vi "Autonomous Independent.vi"   [LabVIEW 2020]
doc: "This VI is called when autonomous begins, and will automatically be terminated when autonomous ends. You can carry out timed or sensor driven robot movement independently without needing to return to the caller."
uses:
  <vilib>/Rock Robotics/WPI/Utilities/WPI_GetSetVariantRefNum.vi
  Robot Global Data.vi
  <vilib>/Rock Robotics/Network Tables/NT Read Number.vi
  <vilib>/Rock Robotics/Network Tables/NT Write Numeric Array.vi
  <vilib>/Rock Robotics/Network Tables/NT Read String.vi
panel:
  # "Be sure to right-click and choose Data Operations>>Make Current Value default if you want to save the array values with the VI"
types:
  T1 = typedef "WPI_JoystickDevRef.ctl" = cluster{"Device":T2}
  T2 = typedef "WPI_JoystickDeviceEnum.ctl" = enum16{"USB 0", "USB 1", "USB 2", "USB 3", "USB 4", "USB 5"}
  T3 = typedef "WPI_MotorControlDeviceRef.ctl" = cluster{"DeviceStatus":errorcluster, "Type":T4, "PWM":cluster{"PWM Channel":T5, "DeadBand":T6}, "CAN":cluster{"Device Number":u8, "SetOutput VI Ref":variant, "GetOutput VI Ref":variant, "Enable VI Ref":variant, "Disable VI Ref":variant, "Data":variant}, "Invert":bool, "DIO PWM":cluster{"PWM \"Enable\" Channel":T5, "DIOChannel":T7, "PWM Rate":dbl}}
  T4 = typedef "WPI_MotorControlType.ctl" = enum16{"PWM", "CAN", "DIO PWM"}
  T5 = typedef "FPGA_DIOPWMChannel.ctl" = enum8{"PWM 0", "PWM 1", "PWM 2", "PWM 3", "PWM 4", "PWM 5", "PWM 6", "PWM 7", "PWM 8", "PWM 9", "PWM MXP 0", "PWM MXP 1", "PWM MXP 2", "PWM MXP 3", "PWM MXP 4", "PWM MXP 5", "PWM MXP 6", "PWM MXP 7", "PWM MXP 8", "PWM MXP 9", "Invalid"}
  T6 = typedef "WPI_PWMDeadband.ctl" = cluster{"Name":string, "maxPositivePwm":i32, "minPositivePwm":i32, "centerPwm":i32, "maxNegativePwm":i32, "minNegativePwm":i32, "angularRange":u16}
  T7 = typedef "FPGA_DIOChannel.ctl" = enum8{"DIO 0", "DIO 1", "DIO 2", "DIO 3", "DIO 4", "DIO 5", "DIO 6", "DIO 7", "DIO 8", "DIO 9", "DIO MXP 0", "DIO MXP 1", "DIO MXP 2", "DIO MXP 3", "DIO MXP 4", "DIO MXP 5", "DIO MXP 6", "DIO MXP 7", "DIO MXP 8", "DIO MXP 9", "DIO MXP 10", "DIO MXP 11", "DIO MXP 12", "DIO MXP 13", "DIO MXP 14", "DIO MXP 15", "SPI Port CS1", "SPI Port CS2", "SPI Port CS3", "SPI Port MISO", "SPI Port MOSI", "Invalid"}
  T8 = typedef "WPI_RobotDriveDevRef.ctl" = cluster{"DevStatus":errorcluster, "Motors[]":T3[], "Square Inputs":bool, "Max Output":dbl}
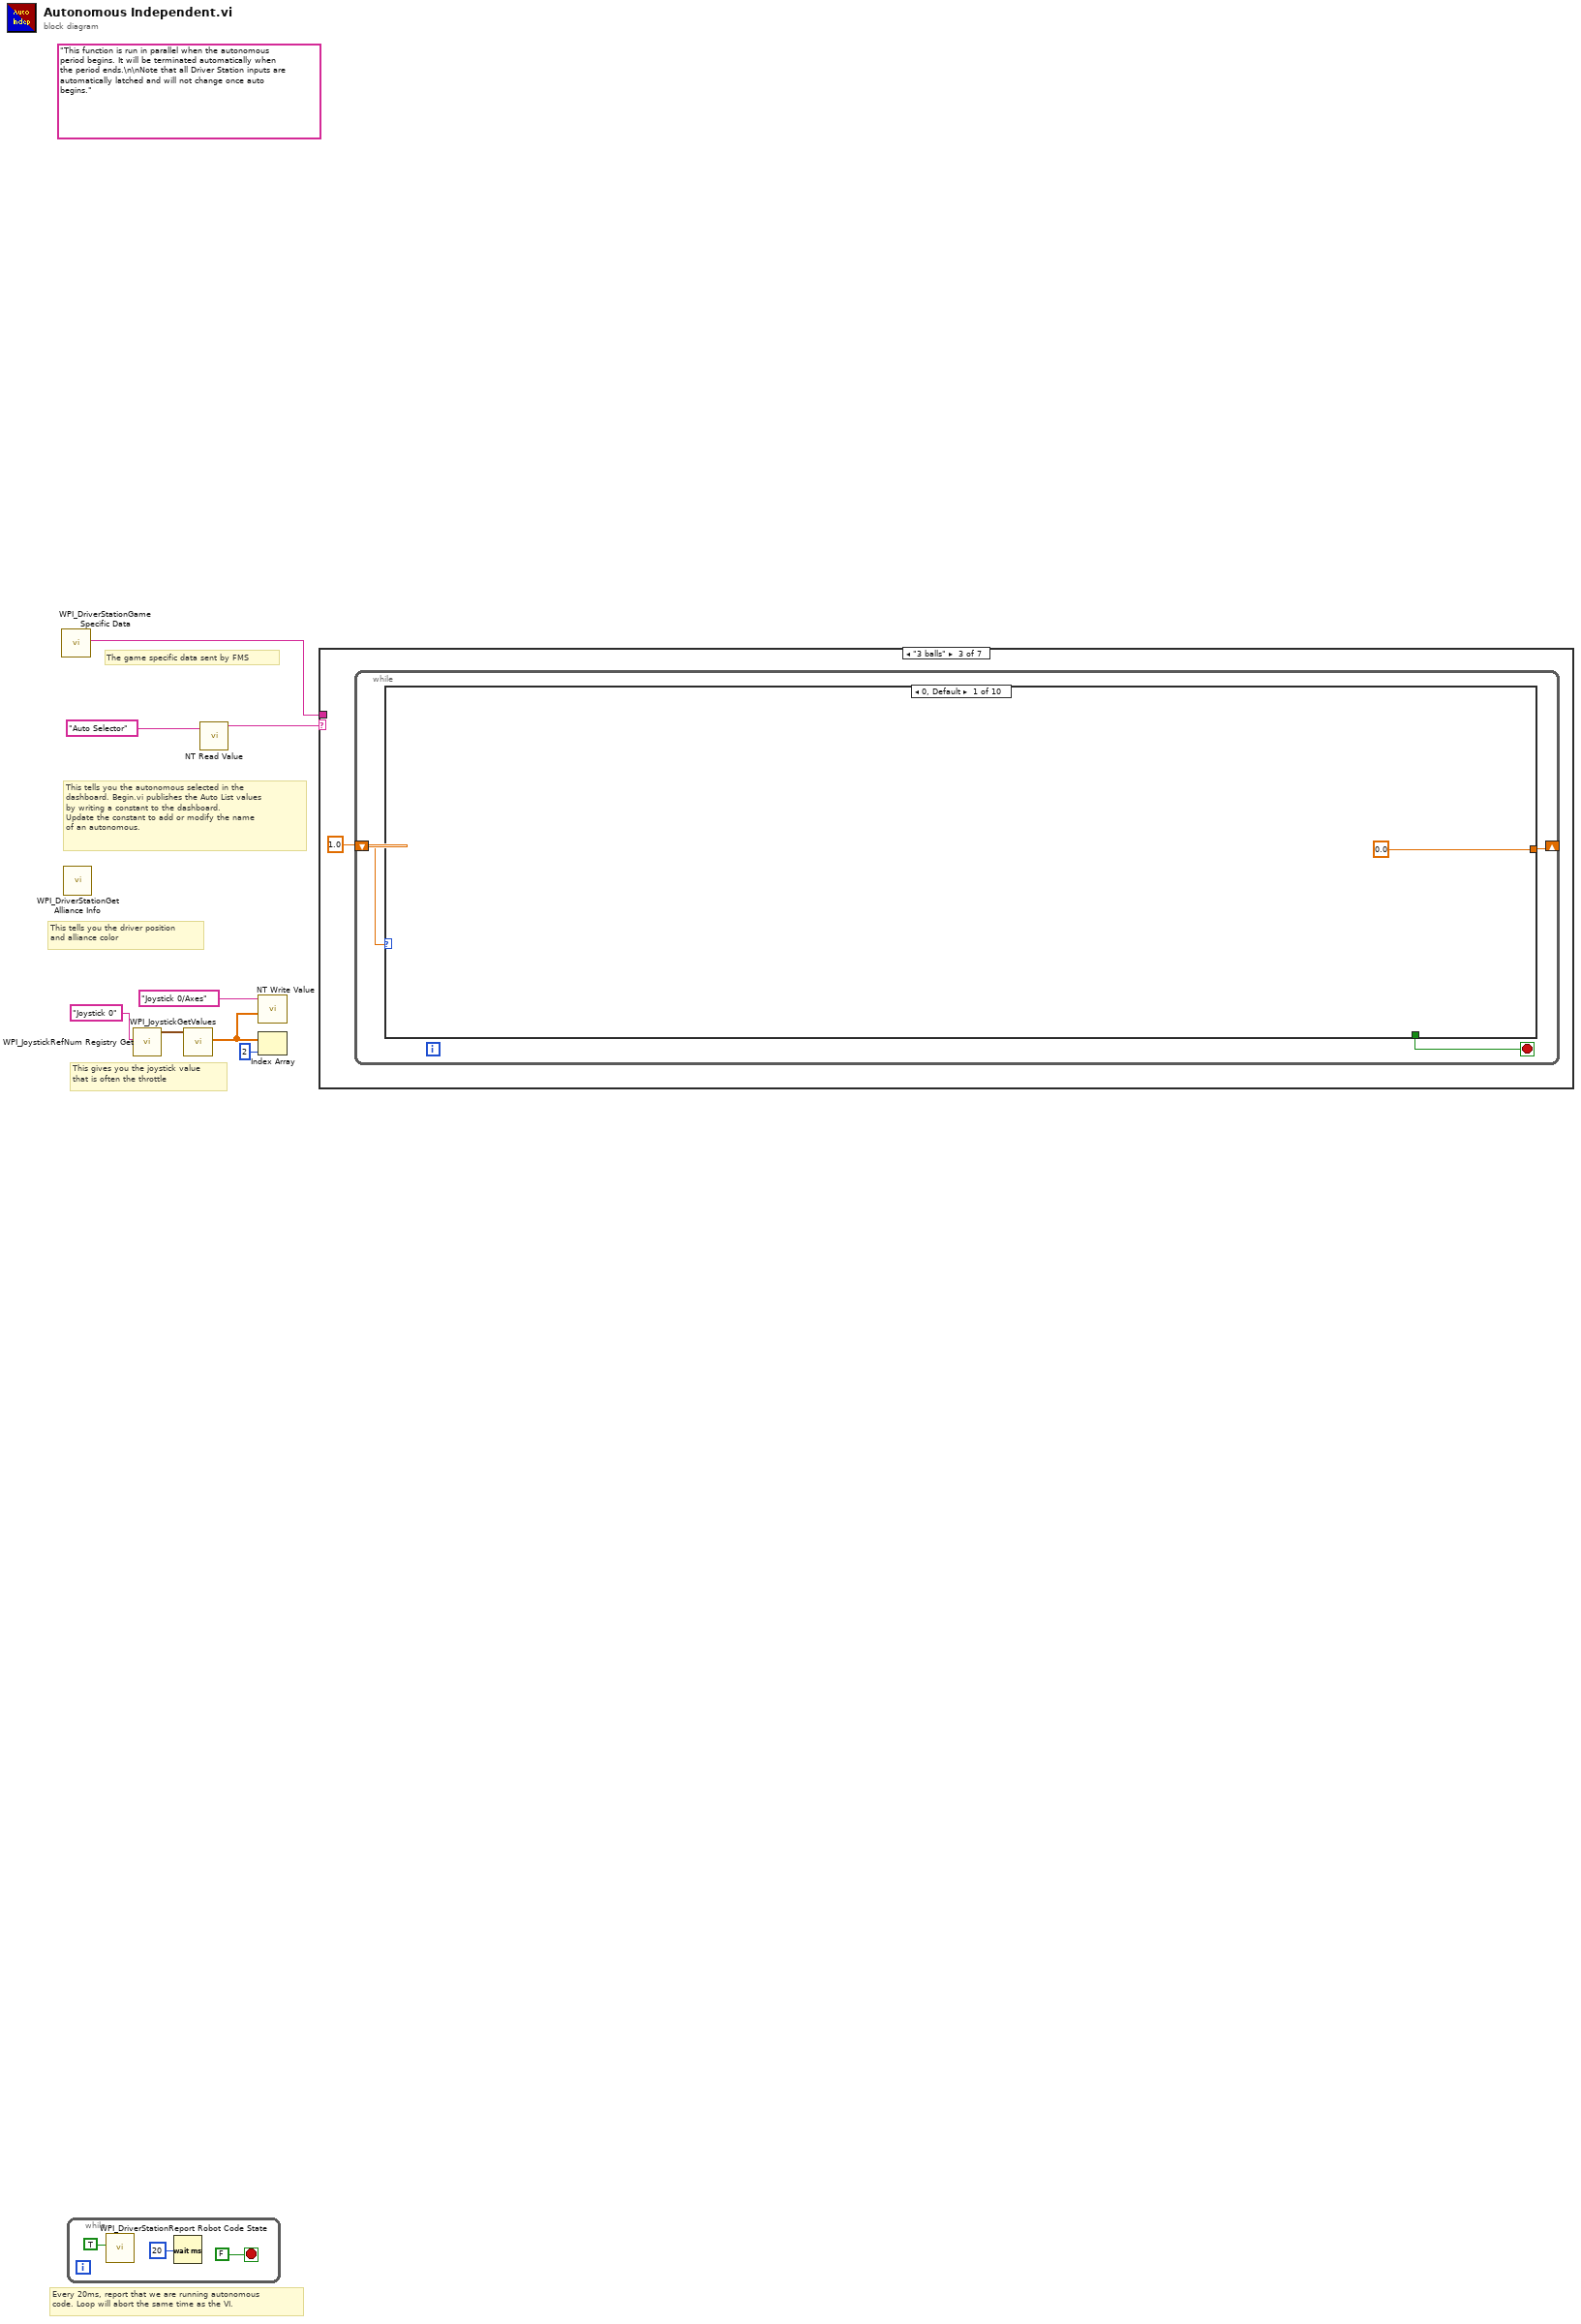
[diagram p0: block diagram]
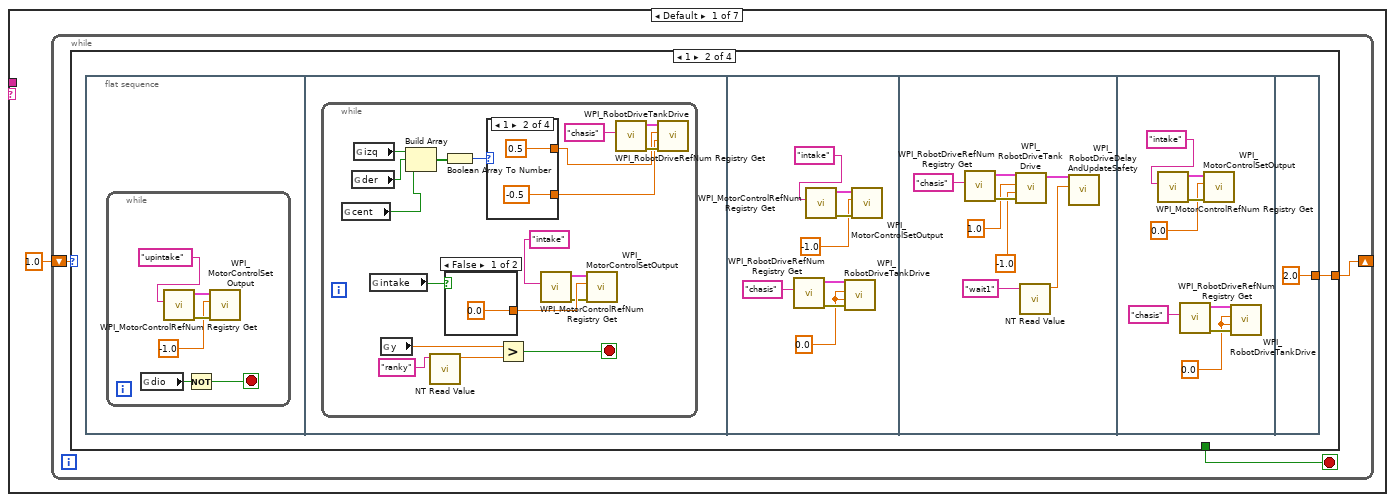
[diagram p2: hidden frame]
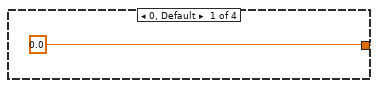
[diagram p3: hidden frame]
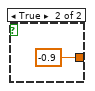
[diagram p4: hidden frame]
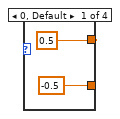
[diagram p5: hidden frame]
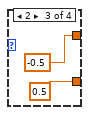
[diagram p6: hidden frame]
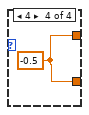
[diagram p7: hidden frame]
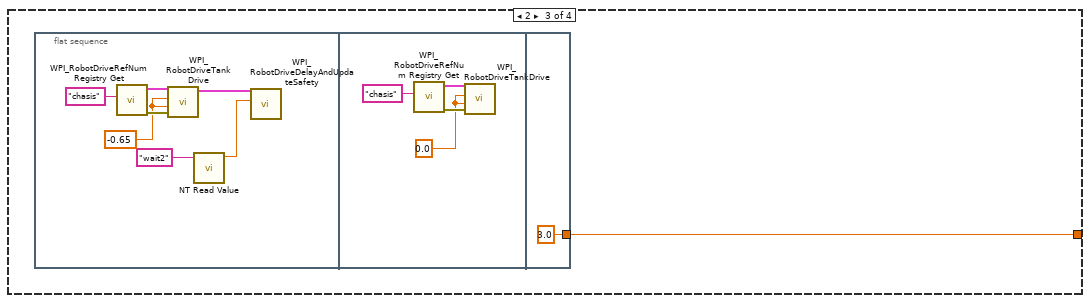
[diagram p8: hidden frame]
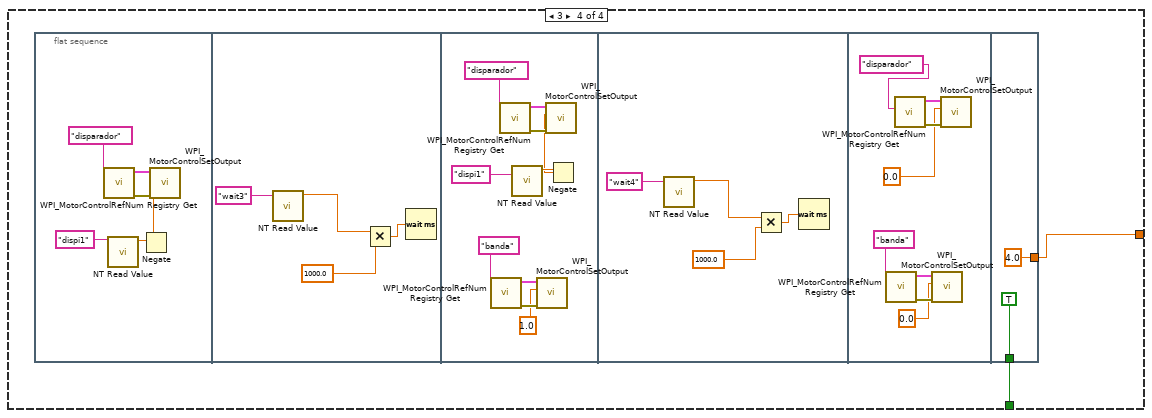
[diagram p9: hidden frame]
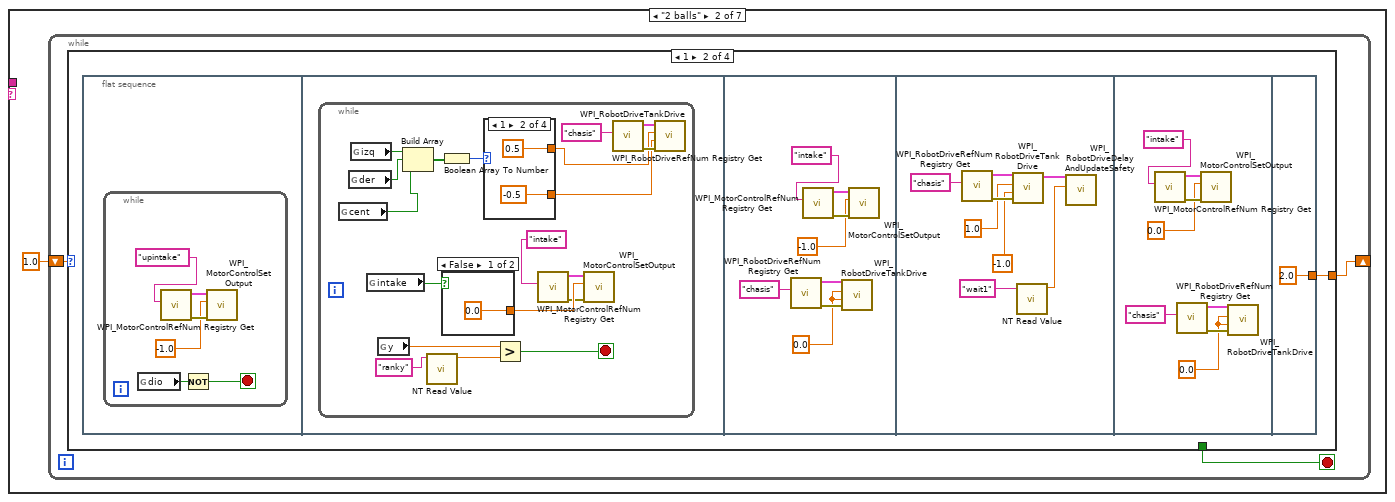
[diagram p10: hidden frame]
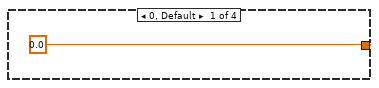
[diagram p11: hidden frame]
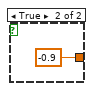
[diagram p12: hidden frame]
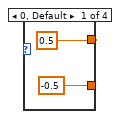
[diagram p13: hidden frame]
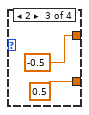
[diagram p14: hidden frame]
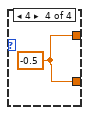
[diagram p15: hidden frame]
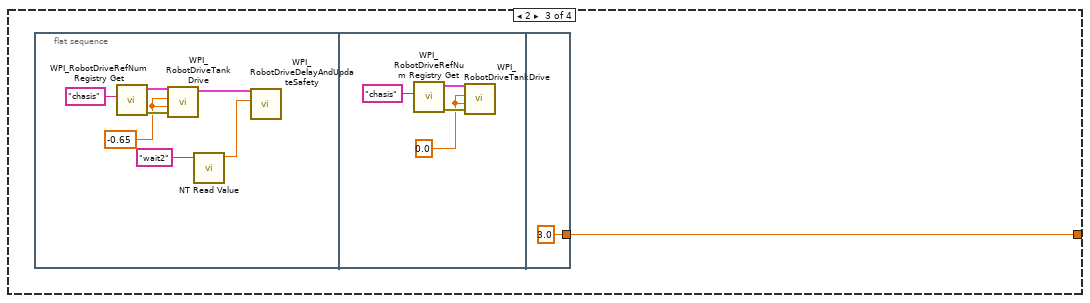
[diagram p16: hidden frame]
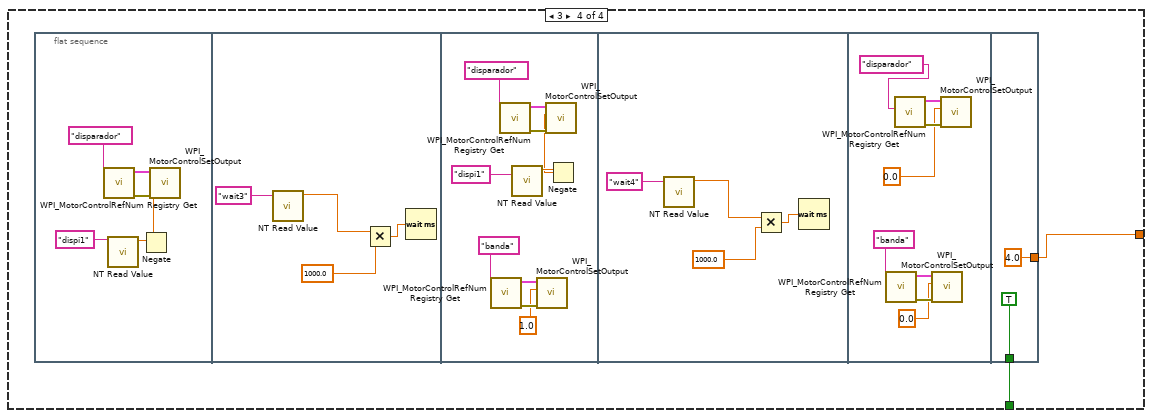
[diagram p17: hidden frame]
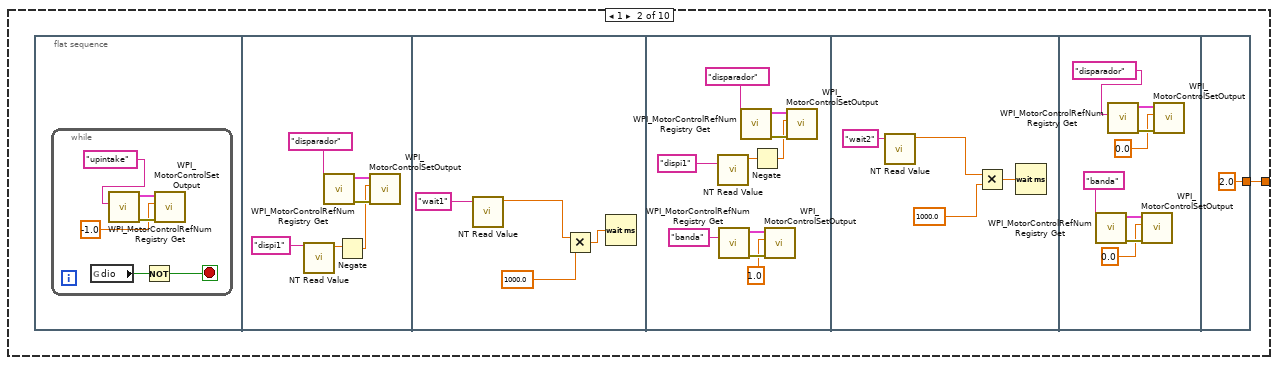
[diagram p18: hidden frame]
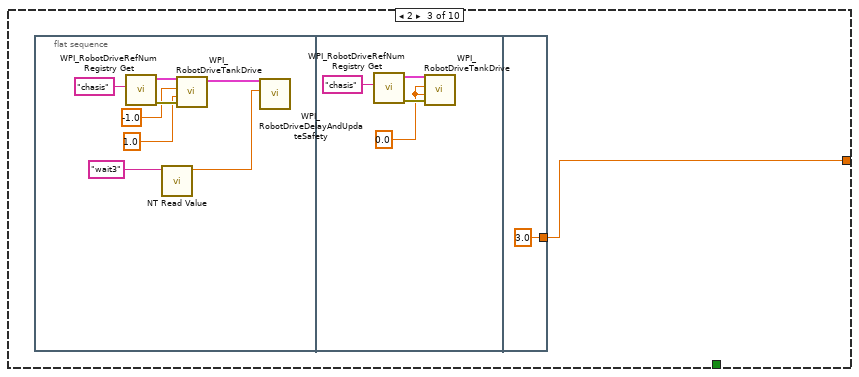
[diagram p19: hidden frame]
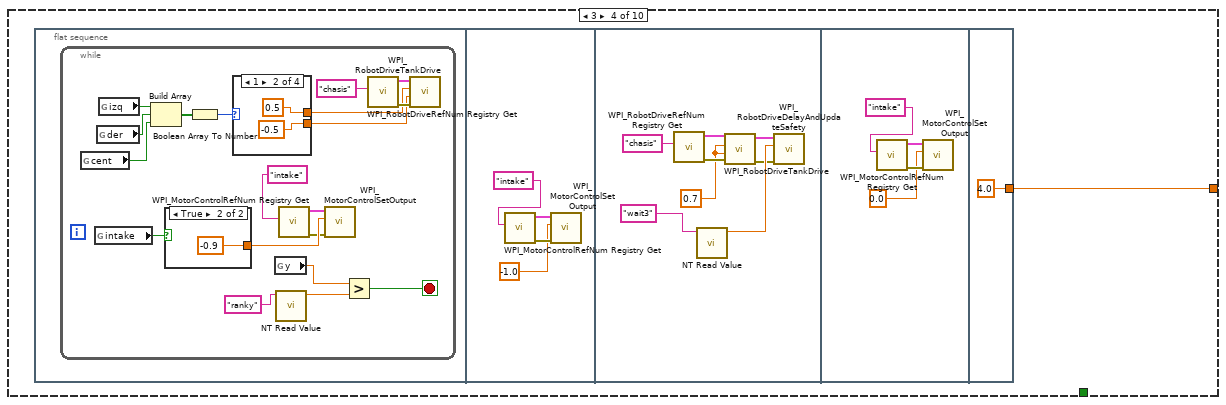
[diagram p20: hidden frame]
diagram:
  (unwired) "This function is run in parallel when the autonomous period begins. It will be terminated automatically when the period ends.\n\nNote that all Driver Station inputs are automatically latched and will not change once auto begins."
  # "The game specific data sent by FMS"
  # "This tells you the autonomous selected in the \ndashboard. Begin.vi publishes the Auto List values\nby writing a constant to the dashboard.\nUpdate the constant to add or modify the name\nof an autonomous."
  # "Every 20ms, report that we are running autonomous\ncode. Loop will abort the same time as the VI."
  # "This gives you the joystick value\nthat is often the throttle"
  # "This tells you the driver position\nand alliance color"
  n1 = call <vilib>:"WPI_DriverStationGame Specific Data.vi"() -> ("Game Specific Data"=w1:string)  [unwired: 11 in]
  n2 = call <vilib>:"WPI_DriverStationGet Alliance Info.vi"() -> ()  [unwired: 12 out]
  n3 = while {
    stop <- FALSE stop-if-true
    n4 = call <vilib>:"WPI_DriverStationReport Robot Code State.vi"("Autonomous"=TRUE) -> ()  [unwired: 10 in, 1 out]
    n5 = Wait (ms)(milliseconds to wait=u32 20) -> ()  [unwired: 1 out]
  }
  n6 = call <vilib>:"WPI_JoystickRefNum Registry Get.vi"("refnum name"="Joystick 0") -> ("JoystickDevRef"=w7:T1)  [unwired: 1 in, 9 out]
  n7 = call <vilib>:"WPI_JoystickGetValues.vi"("JoystickDevRef"=w7) -> ("Axes"=w3:dbl[])  [unwired: 6 in, 4 out]
  n8 = call-poly <vilib>:"NT Read Value.vi"("Name"="Auto Selector") -> ("String"=w4:string)  [unwired: 9 in, 1 out]
  n9 = call-poly <vilib>:"NT Write Value.vi"("Numeric Array"=w3, "Name"="Joystick 0/Axes") -> ()  [unwired: 9 in, 1 out]
  n10 = Index Array(array=w3, index=2) -> ()  [unwired: 1 out]
  n11 = case shown="\"3 balls\"" w4 {
    tunnel: w1 -> [_ _ _ _ _ _ _]
    frame Default {
      n12 = while {
        shift-right: [w14] -> _
        shift-left: 1.0 -> [w15]
        stop <- w13 stop-if-true
        n13 = case shown="1" w15 {
          tunnel: [0.0 w17 w77 w90] -> w14
          tunnel: [_ _ _ w91] -> w13
          frame 0, Default {
          }
          frame 1 {
            n14 = flat-sequence {
              tunnel: [2.0] -> w17
              frame #0 {
                n15 = while {
                  stop <- w18 stop-if-true
                  n16 = global read "Robot Global Data.vi" "dio"() -> (w19:bool)
                  n17 = call <vilib>:"WPI_MotorControlRefNum Registry Get.vi"("refnum name"="upintake") -> ("error out"=w22:errorcluster, "MotorControlDevRef"=w23:T3)  [unwired: 9 in]
                  n18 = Not(x=w19) -> (.not. x?=w18:bool)
                  n19 = call <vilib>:"WPI_MotorControlSetOutput.vi"("error in (no error)"=w22, "Output"=-1.0, "MotorControlDevRef"=w23) -> ()  [unwired: 6 in, 3 out]
                }
              }
              frame #1 {
                n20 = while {
                  stop <- w27 stop-if-true
                  n21 = global read "Robot Global Data.vi" "cent"() -> (w28:bool)
                  n22 = global read "Robot Global Data.vi" "der"() -> (w41:bool)
                  n23 = global read "Robot Global Data.vi" "izq"() -> (w42:bool)
                  n24 = global read "Robot Global Data.vi" "intake"() -> (w25:bool)
                  n25 = global read "Robot Global Data.vi" "y"() -> (w26:dbl)
                  n26 = Build Array(w42, w41, w28) -> (w40:bool[])
                  n27 = call-poly <vilib>:"NT Read Value.vi"("Name"="ranky") -> ("Numeric"=w24:dbl)  [unwired: 9 in, 1 out]
                  n28 = Boolean Array To Number(Boolean array=w40) -> (number=w39:u32)
                  n29 = case shown="False" w25 {
                    tunnel: [0.0 -0.9] -> w33
                    frame False {
                    }
                    frame True {
                    }
                  }
                  n30 = case shown="1" w39 {
                    tunnel: [0.5 0.5 -0.5 w51] -> w35
                    tunnel: [-0.5 -0.5 0.5 w51] -> w34
                    frame 0, Default {
                    }
                    frame 1 {
                    }
                    frame 2 {
                    }
                    frame 4 {
                      w51 = -0.5
                    }
                  }
                  n31 = Greater?(x=w26, y=w24) -> (0:w27:bool)
                  n32 = call <vilib>:"WPI_MotorControlRefNum Registry Get.vi"("refnum name"="intake") -> ("error out"=w31:errorcluster, "MotorControlDevRef"=w32:T3)  [unwired: 9 in]
                  n33 = call <vilib>:"WPI_MotorControlSetOutput.vi"("error in (no error)"=w31, "Output"=w33, "MotorControlDevRef"=w32) -> ()  [unwired: 6 in, 3 out]
                  n34 = call <vilib>:"WPI_RobotDriveRefNum Registry Get.vi"("refnum name"="chasis") -> ("error out"=w37:errorcluster, "RobotDriveDevRef"=w38:T8)  [unwired: 9 in]
                  n35 = call <vilib>:"WPI_RobotDriveTankDrive.vi"("error in (no error)"=w37, "Right axis value"=w34, "Left axis value"=w35, "RobotDriveDevRef"=w38) -> ()  [unwired: 5 in, 3 out]
                }
              }
              frame #2 {
                w56 = 0.0
                n36 = call <vilib>:"WPI_RobotDriveRefNum Registry Get.vi"("refnum name"="chasis") -> ("error out"=w57:errorcluster, "RobotDriveDevRef"=w58:T8)  [unwired: 9 in]
                n37 = call <vilib>:"WPI_MotorControlRefNum Registry Get.vi"("refnum name"="intake") -> ("error out"=w55:errorcluster, "MotorControlDevRef"=w54:T3)  [unwired: 9 in]
                n38 = call <vilib>:"WPI_RobotDriveTankDrive.vi"("error in (no error)"=w57, "Right axis value"=w56, "Left axis value"=w56, "RobotDriveDevRef"=w58) -> ()  [unwired: 5 in, 3 out]
                n39 = call <vilib>:"WPI_MotorControlSetOutput.vi"("error in (no error)"=w55, "Output"=-1.0, "MotorControlDevRef"=w54) -> ()  [unwired: 6 in, 3 out]
              }
              frame #3 {
                n40 = call <vilib>:"WPI_RobotDriveRefNum Registry Get.vi"("refnum name"="chasis") -> ("error out"=w67:errorcluster, "RobotDriveDevRef"=w66:T8)  [unwired: 9 in]
                n41 = call <vilib>:"WPI_RobotDriveTankDrive.vi"("error in (no error)"=w67, "Right axis value"=-1.0, "Left axis value"=1.0, "RobotDriveDevRef"=w66) -> ("RobotDriveDevRef"=w61:T8)  [unwired: 5 in, 2 out]
                n42 = call-poly <vilib>:"NT Read Value.vi"("Name"="wait1") -> ("Numeric"=w60:dbl)  [unwired: 9 in, 1 out]
                n43 = call <vilib>:"WPI_RobotDriveDelayAndUpdateSafety.vi"("Delay (s)"=w60, "RobotDriveDevRef"=w61) -> ()  [unwired: 8 in, 2 out]
              }
              frame #4 {
                w72 = 0.0
                n44 = call <vilib>:"WPI_MotorControlRefNum Registry Get.vi"("refnum name"="intake") -> ("error out"=w70:errorcluster, "MotorControlDevRef"=w71:T3)  [unwired: 9 in]
                n45 = call <vilib>:"WPI_RobotDriveRefNum Registry Get.vi"("refnum name"="chasis") -> ("error out"=w73:errorcluster, "RobotDriveDevRef"=w74:T8)  [unwired: 9 in]
                n46 = call <vilib>:"WPI_MotorControlSetOutput.vi"("error in (no error)"=w70, "Output"=0.0, "MotorControlDevRef"=w71) -> ()  [unwired: 6 in, 3 out]
                n47 = call <vilib>:"WPI_RobotDriveTankDrive.vi"("error in (no error)"=w73, "Right axis value"=w72, "Left axis value"=w72, "RobotDriveDevRef"=w74) -> ()  [unwired: 5 in, 3 out]
              }
              frame #5 {
              }
            }
          }
          frame 2 {
            n48 = flat-sequence {
              tunnel: [3.0] -> w77
              frame #0 {
                w78 = -0.65 ("Left axis value")
                n49 = call <vilib>:"WPI_RobotDriveRefNum Registry Get.vi"("refnum name"="chasis") -> ("error out"=w84:errorcluster, "RobotDriveDevRef"=w83:T8)  [unwired: 9 in]
                n50 = call <vilib>:"WPI_RobotDriveTankDrive.vi"("error in (no error)"=w84, "Right axis value"=w78, "Left axis value"=w78, "RobotDriveDevRef"=w83) -> ("RobotDriveDevRef"=w80:T8)  [unwired: 5 in, 2 out]
                n51 = call-poly <vilib>:"NT Read Value.vi"("Name"="wait2") -> ("Numeric"=w79:dbl)  [unwired: 9 in, 1 out]
                n52 = call <vilib>:"WPI_RobotDriveDelayAndUpdateSafety.vi"("Delay (s)"=w79, "RobotDriveDevRef"=w80) -> ()  [unwired: 8 in, 2 out]
              }
              frame #1 {
                w85 = 0.0
                n53 = call <vilib>:"WPI_RobotDriveRefNum Registry Get.vi"("refnum name"="chasis") -> ("error out"=w86:errorcluster, "RobotDriveDevRef"=w87:T8)  [unwired: 9 in]
                n54 = call <vilib>:"WPI_RobotDriveTankDrive.vi"("error in (no error)"=w86, "Right axis value"=w85, "Left axis value"=w85, "RobotDriveDevRef"=w87) -> ()  [unwired: 5 in, 3 out]
              }
              frame #2 {
              }
            }
          }
          frame 3 {
            n55 = flat-sequence {
              tunnel: [TRUE] -> w91
              tunnel: [4.0] -> w90
              frame #0 {
                n56 = call <vilib>:"WPI_MotorControlRefNum Registry Get.vi"("refnum name"="disparador") -> ("error out"=w97:errorcluster, "MotorControlDevRef"=w96:T3)  [unwired: 9 in]
                n57 = call-poly <vilib>:"NT Read Value.vi"("Name"="dispi1") -> ("Numeric"=w93:dbl)  [unwired: 9 in, 1 out]
                n58 = Negate(x=w93) -> (-x=w92:dbl)
                n59 = call <vilib>:"WPI_MotorControlSetOutput.vi"("error in (no error)"=w97, "Output"=w92, "MotorControlDevRef"=w96) -> ()  [unwired: 6 in, 3 out]
              }
              frame #1 {
                n60 = call-poly <vilib>:"NT Read Value.vi"("Name"="wait3") -> ("Numeric"=w100:dbl)  [unwired: 9 in, 1 out]
                n61 = Multiply(x=w100, y=1000.0) -> (x*y=w101:dbl)
                n62 = Wait (ms)(milliseconds to wait=w101) -> ()  [unwired: 1 out]
              }
              frame #2 {
                n63 = call <vilib>:"WPI_MotorControlRefNum Registry Get.vi"("refnum name"="banda") -> ("error out"=w107:errorcluster, "MotorControlDevRef"=w106:T3)  [unwired: 9 in]
                n64 = call <vilib>:"WPI_MotorControlRefNum Registry Get.vi"("refnum name"="disparador") -> ("error out"=w111:errorcluster, "MotorControlDevRef"=w110:T3)  [unwired: 9 in]
                n65 = call-poly <vilib>:"NT Read Value.vi"("Name"="dispi1") -> ("Numeric"=w103:dbl)  [unwired: 9 in, 1 out]
                n66 = call <vilib>:"WPI_MotorControlSetOutput.vi"("error in (no error)"=w107, "Output"=1.0, "MotorControlDevRef"=w106) -> ()  [unwired: 6 in, 3 out]
                n67 = Negate(x=w103) -> (-x=w102:dbl)
                n68 = call <vilib>:"WPI_MotorControlSetOutput.vi"("error in (no error)"=w111, "Output"=w102, "MotorControlDevRef"=w110) -> ()  [unwired: 6 in, 3 out]
              }
              frame #3 {
                n69 = call-poly <vilib>:"NT Read Value.vi"("Name"="wait4") -> ("Numeric"=w115:dbl)  [unwired: 9 in, 1 out]
                n70 = Multiply(x=w115, y=1000.0) -> (x*y=w112:dbl)
                n71 = Wait (ms)(milliseconds to wait=w112) -> ()  [unwired: 1 out]
              }
              frame #4 {
                n72 = call <vilib>:"WPI_MotorControlRefNum Registry Get.vi"("refnum name"="banda") -> ("error out"=w121:errorcluster, "MotorControlDevRef"=w120:T3)  [unwired: 9 in]
                n73 = call <vilib>:"WPI_MotorControlRefNum Registry Get.vi"("refnum name"="disparador") -> ("error out"=w123:errorcluster, "MotorControlDevRef"=w122:T3)  [unwired: 9 in]
                n74 = call <vilib>:"WPI_MotorControlSetOutput.vi"("error in (no error)"=w121, "Output"=0.0, "MotorControlDevRef"=w120) -> ()  [unwired: 6 in, 3 out]
                n75 = call <vilib>:"WPI_MotorControlSetOutput.vi"("error in (no error)"=w123, "Output"=0.0, "MotorControlDevRef"=w122) -> ()  [unwired: 6 in, 3 out]
              }
              frame #5 {
              }
            }
          }
        }
      }
    }
    frame "2 balls" {
      n76 = while {
        shift-right: [w128] -> _
        shift-left: 1.0 -> [w129]
        stop <- w127 stop-if-true
        n77 = case shown="1" w129 {
          tunnel: [0.0 w131 w191 w204] -> w128
          tunnel: [_ _ _ w205] -> w127
          frame 0, Default {
          }
          frame 1 {
            n78 = flat-sequence {
              tunnel: [2.0] -> w131
              frame #0 {
                n79 = while {
                  stop <- w132 stop-if-true
                  n80 = global read "Robot Global Data.vi" "dio"() -> (w133:bool)
                  n81 = call <vilib>:"WPI_MotorControlRefNum Registry Get.vi"("refnum name"="upintake") -> ("error out"=w136:errorcluster, "MotorControlDevRef"=w137:T3)  [unwired: 9 in]
                  n82 = Not(x=w133) -> (.not. x?=w132:bool)
                  n83 = call <vilib>:"WPI_MotorControlSetOutput.vi"("error in (no error)"=w136, "Output"=-1.0, "MotorControlDevRef"=w137) -> ()  [unwired: 6 in, 3 out]
                }
              }
              frame #1 {
                n84 = while {
                  stop <- w141 stop-if-true
                  n85 = global read "Robot Global Data.vi" "cent"() -> (w142:bool)
                  n86 = global read "Robot Global Data.vi" "der"() -> (w155:bool)
                  n87 = global read "Robot Global Data.vi" "izq"() -> (w156:bool)
                  n88 = global read "Robot Global Data.vi" "intake"() -> (w139:bool)
                  n89 = global read "Robot Global Data.vi" "y"() -> (w140:dbl)
                  n90 = Build Array(w156, w155, w142) -> (w154:bool[])
                  n91 = call-poly <vilib>:"NT Read Value.vi"("Name"="ranky") -> ("Numeric"=w138:dbl)  [unwired: 9 in, 1 out]
                  n92 = Boolean Array To Number(Boolean array=w154) -> (number=w153:u32)
                  n93 = case shown="False" w139 {
                    tunnel: [0.0 -0.9] -> w147
                    frame False {
                    }
                    frame True {
                    }
                  }
                  n94 = case shown="1" w153 {
                    tunnel: [0.5 0.5 -0.5 w165] -> w149
                    tunnel: [-0.5 -0.5 0.5 w165] -> w148
                    frame 0, Default {
                    }
                    frame 1 {
                    }
                    frame 2 {
                    }
                    frame 4 {
                      w165 = -0.5
                    }
                  }
                  n95 = Greater?(x=w140, y=w138) -> (0:w141:bool)
                  n96 = call <vilib>:"WPI_MotorControlRefNum Registry Get.vi"("refnum name"="intake") -> ("error out"=w145:errorcluster, "MotorControlDevRef"=w146:T3)  [unwired: 9 in]
                  n97 = call <vilib>:"WPI_MotorControlSetOutput.vi"("error in (no error)"=w145, "Output"=w147, "MotorControlDevRef"=w146) -> ()  [unwired: 6 in, 3 out]
                  n98 = call <vilib>:"WPI_RobotDriveRefNum Registry Get.vi"("refnum name"="chasis") -> ("error out"=w151:errorcluster, "RobotDriveDevRef"=w152:T8)  [unwired: 9 in]
                  n99 = call <vilib>:"WPI_RobotDriveTankDrive.vi"("error in (no error)"=w151, "Right axis value"=w148, "Left axis value"=w149, "RobotDriveDevRef"=w152) -> ()  [unwired: 5 in, 3 out]
                }
              }
              frame #2 {
                w170 = 0.0
                n100 = call <vilib>:"WPI_RobotDriveRefNum Registry Get.vi"("refnum name"="chasis") -> ("error out"=w171:errorcluster, "RobotDriveDevRef"=w172:T8)  [unwired: 9 in]
                n101 = call <vilib>:"WPI_MotorControlRefNum Registry Get.vi"("refnum name"="intake") -> ("error out"=w169:errorcluster, "MotorControlDevRef"=w168:T3)  [unwired: 9 in]
                n102 = call <vilib>:"WPI_RobotDriveTankDrive.vi"("error in (no error)"=w171, "Right axis value"=w170, "Left axis value"=w170, "RobotDriveDevRef"=w172) -> ()  [unwired: 5 in, 3 out]
                n103 = call <vilib>:"WPI_MotorControlSetOutput.vi"("error in (no error)"=w169, "Output"=-1.0, "MotorControlDevRef"=w168) -> ()  [unwired: 6 in, 3 out]
              }
              frame #3 {
                n104 = call <vilib>:"WPI_RobotDriveRefNum Registry Get.vi"("refnum name"="chasis") -> ("error out"=w181:errorcluster, "RobotDriveDevRef"=w180:T8)  [unwired: 9 in]
                n105 = call <vilib>:"WPI_RobotDriveTankDrive.vi"("error in (no error)"=w181, "Right axis value"=-1.0, "Left axis value"=1.0, "RobotDriveDevRef"=w180) -> ("RobotDriveDevRef"=w175:T8)  [unwired: 5 in, 2 out]
                n106 = call-poly <vilib>:"NT Read Value.vi"("Name"="wait1") -> ("Numeric"=w174:dbl)  [unwired: 9 in, 1 out]
                n107 = call <vilib>:"WPI_RobotDriveDelayAndUpdateSafety.vi"("Delay (s)"=w174, "RobotDriveDevRef"=w175) -> ()  [unwired: 8 in, 2 out]
              }
              frame #4 {
                w186 = 0.0
                n108 = call <vilib>:"WPI_MotorControlRefNum Registry Get.vi"("refnum name"="intake") -> ("error out"=w184:errorcluster, "MotorControlDevRef"=w185:T3)  [unwired: 9 in]
                n109 = call <vilib>:"WPI_RobotDriveRefNum Registry Get.vi"("refnum name"="chasis") -> ("error out"=w187:errorcluster, "RobotDriveDevRef"=w188:T8)  [unwired: 9 in]
                n110 = call <vilib>:"WPI_MotorControlSetOutput.vi"("error in (no error)"=w184, "Output"=0.0, "MotorControlDevRef"=w185) -> ()  [unwired: 6 in, 3 out]
                n111 = call <vilib>:"WPI_RobotDriveTankDrive.vi"("error in (no error)"=w187, "Right axis value"=w186, "Left axis value"=w186, "RobotDriveDevRef"=w188) -> ()  [unwired: 5 in, 3 out]
              }
              frame #5 {
              }
            }
          }
          frame 2 {
            n112 = flat-sequence {
              tunnel: [3.0] -> w191
              frame #0 {
                w192 = -0.65 ("Left axis value")
                n113 = call <vilib>:"WPI_RobotDriveRefNum Registry Get.vi"("refnum name"="chasis") -> ("error out"=w198:errorcluster, "RobotDriveDevRef"=w197:T8)  [unwired: 9 in]
                n114 = call <vilib>:"WPI_RobotDriveTankDrive.vi"("error in (no error)"=w198, "Right axis value"=w192, "Left axis value"=w192, "RobotDriveDevRef"=w197) -> ("RobotDriveDevRef"=w194:T8)  [unwired: 5 in, 2 out]
                n115 = call-poly <vilib>:"NT Read Value.vi"("Name"="wait2") -> ("Numeric"=w193:dbl)  [unwired: 9 in, 1 out]
                n116 = call <vilib>:"WPI_RobotDriveDelayAndUpdateSafety.vi"("Delay (s)"=w193, "RobotDriveDevRef"=w194) -> ()  [unwired: 8 in, 2 out]
              }
              frame #1 {
                w199 = 0.0
                n117 = call <vilib>:"WPI_RobotDriveRefNum Registry Get.vi"("refnum name"="chasis") -> ("error out"=w200:errorcluster, "RobotDriveDevRef"=w201:T8)  [unwired: 9 in]
                n118 = call <vilib>:"WPI_RobotDriveTankDrive.vi"("error in (no error)"=w200, "Right axis value"=w199, "Left axis value"=w199, "RobotDriveDevRef"=w201) -> ()  [unwired: 5 in, 3 out]
              }
              frame #2 {
              }
            }
          }
          frame 3 {
            n119 = flat-sequence {
              tunnel: [TRUE] -> w205
              tunnel: [4.0] -> w204
              frame #0 {
                n120 = call <vilib>:"WPI_MotorControlRefNum Registry Get.vi"("refnum name"="disparador") -> ("error out"=w211:errorcluster, "MotorControlDevRef"=w210:T3)  [unwired: 9 in]
                n121 = call-poly <vilib>:"NT Read Value.vi"("Name"="dispi1") -> ("Numeric"=w207:dbl)  [unwired: 9 in, 1 out]
                n122 = Negate(x=w207) -> (-x=w206:dbl)
                n123 = call <vilib>:"WPI_MotorControlSetOutput.vi"("error in (no error)"=w211, "Output"=w206, "MotorControlDevRef"=w210) -> ()  [unwired: 6 in, 3 out]
              }
              frame #1 {
                n124 = call-poly <vilib>:"NT Read Value.vi"("Name"="wait3") -> ("Numeric"=w214:dbl)  [unwired: 9 in, 1 out]
                n125 = Multiply(x=w214, y=1000.0) -> (x*y=w215:dbl)
                n126 = Wait (ms)(milliseconds to wait=w215) -> ()  [unwired: 1 out]
              }
              frame #2 {
                n127 = call <vilib>:"WPI_MotorControlRefNum Registry Get.vi"("refnum name"="banda") -> ("error out"=w221:errorcluster, "MotorControlDevRef"=w220:T3)  [unwired: 9 in]
                n128 = call <vilib>:"WPI_MotorControlRefNum Registry Get.vi"("refnum name"="disparador") -> ("error out"=w225:errorcluster, "MotorControlDevRef"=w224:T3)  [unwired: 9 in]
                n129 = call-poly <vilib>:"NT Read Value.vi"("Name"="dispi1") -> ("Numeric"=w217:dbl)  [unwired: 9 in, 1 out]
                n130 = call <vilib>:"WPI_MotorControlSetOutput.vi"("error in (no error)"=w221, "Output"=1.0, "MotorControlDevRef"=w220) -> ()  [unwired: 6 in, 3 out]
                n131 = Negate(x=w217) -> (-x=w216:dbl)
                n132 = call <vilib>:"WPI_MotorControlSetOutput.vi"("error in (no error)"=w225, "Output"=w216, "MotorControlDevRef"=w224) -> ()  [unwired: 6 in, 3 out]
              }
              frame #3 {
                n133 = call-poly <vilib>:"NT Read Value.vi"("Name"="wait4") -> ("Numeric"=w229:dbl)  [unwired: 9 in, 1 out]
                n134 = Multiply(x=w229, y=1000.0) -> (x*y=w226:dbl)
                n135 = Wait (ms)(milliseconds to wait=w226) -> ()  [unwired: 1 out]
              }
              frame #4 {
                n136 = call <vilib>:"WPI_MotorControlRefNum Registry Get.vi"("refnum name"="banda") -> ("error out"=w235:errorcluster, "MotorControlDevRef"=w234:T3)  [unwired: 9 in]
                n137 = call <vilib>:"WPI_MotorControlRefNum Registry Get.vi"("refnum name"="disparador") -> ("error out"=w237:errorcluster, "MotorControlDevRef"=w236:T3)  [unwired: 9 in]
                n138 = call <vilib>:"WPI_MotorControlSetOutput.vi"("error in (no error)"=w235, "Output"=0.0, "MotorControlDevRef"=w234) -> ()  [unwired: 6 in, 3 out]
                n139 = call <vilib>:"WPI_MotorControlSetOutput.vi"("error in (no error)"=w237, "Output"=0.0, "MotorControlDevRef"=w236) -> ()  [unwired: 6 in, 3 out]
              }
              frame #5 {
              }
            }
          }
        }
      }
    }
    frame "3 balls" {
      n140 = while {
        shift-right: [w243] -> _
        shift-left: 1.0 -> [w241]
        stop <- w242 stop-if-true
        n141 = case shown="0, Default" w241 {
          tunnel: [0.0 w245 w285 w299 w344 w362 w408 w421 w435 w449] -> w243
          tunnel: [_ _ _ _ _ _ _ _ _ w448] -> w242
          frame 0, Default {
          }
          frame 1 {
            n142 = flat-sequence {
              tunnel: [2.0] -> w245
              frame #0 {
                n143 = while {
                  stop <- w246 stop-if-true
                  n144 = global read "Robot Global Data.vi" "dio"() -> (w247:bool)
                  n145 = call <vilib>:"WPI_MotorControlRefNum Registry Get.vi"("refnum name"="upintake") -> ("error out"=w250:errorcluster, "MotorControlDevRef"=w251:T3)  [unwired: 9 in]
                  n146 = Not(x=w247) -> (.not. x?=w246:bool)
                  n147 = call <vilib>:"WPI_MotorControlSetOutput.vi"("error in (no error)"=w250, "Output"=-1.0, "MotorControlDevRef"=w251) -> ()  [unwired: 6 in, 3 out]
                }
              }
              frame #1 {
                n148 = call-poly <vilib>:"NT Read Value.vi"("Name"="dispi1") -> ("Numeric"=w253:dbl)  [unwired: 9 in, 1 out]
                n149 = call <vilib>:"WPI_MotorControlRefNum Registry Get.vi"("refnum name"="disparador") -> ("error out"=w257:errorcluster, "MotorControlDevRef"=w256:T3)  [unwired: 9 in]
                n150 = Negate(x=w253) -> (-x=w252:dbl)
                n151 = call <vilib>:"WPI_MotorControlSetOutput.vi"("error in (no error)"=w257, "Output"=w252, "MotorControlDevRef"=w256) -> ()  [unwired: 6 in, 3 out]
              }
              frame #2 {
                n152 = call-poly <vilib>:"NT Read Value.vi"("Name"="wait1") -> ("Numeric"=w260:dbl)  [unwired: 9 in, 1 out]
                n153 = Multiply(x=w260, y=1000.0) -> (x*y=w261:dbl)
                n154 = Wait (ms)(milliseconds to wait=w261) -> ()  [unwired: 1 out]
              }
              frame #3 {
                n155 = call-poly <vilib>:"NT Read Value.vi"("Name"="dispi1") -> ("Numeric"=w262:dbl)  [unwired: 9 in, 1 out]
                n156 = call <vilib>:"WPI_MotorControlRefNum Registry Get.vi"("refnum name"="banda") -> ("error out"=w267:errorcluster, "MotorControlDevRef"=w266:T3)  [unwired: 9 in]
                n157 = call <vilib>:"WPI_MotorControlRefNum Registry Get.vi"("refnum name"="disparador") -> ("error out"=w271:errorcluster, "MotorControlDevRef"=w270:T3)  [unwired: 9 in]
                n158 = Negate(x=w262) -> (-x=w263:dbl)
                n159 = call <vilib>:"WPI_MotorControlSetOutput.vi"("error in (no error)"=w267, "Output"=1.0, "MotorControlDevRef"=w266) -> ()  [unwired: 6 in, 3 out]
                n160 = call <vilib>:"WPI_MotorControlSetOutput.vi"("error in (no error)"=w271, "Output"=w263, "MotorControlDevRef"=w270) -> ()  [unwired: 6 in, 3 out]
              }
              frame #4 {
                n161 = call-poly <vilib>:"NT Read Value.vi"("Name"="wait2") -> ("Numeric"=w275:dbl)  [unwired: 9 in, 1 out]
                n162 = Multiply(x=w275, y=1000.0) -> (x*y=w272:dbl)
                n163 = Wait (ms)(milliseconds to wait=w272) -> ()  [unwired: 1 out]
              }
              frame #5 {
                n164 = call <vilib>:"WPI_MotorControlRefNum Registry Get.vi"("refnum name"="banda") -> ("error out"=w281:errorcluster, "MotorControlDevRef"=w280:T3)  [unwired: 9 in]
                n165 = call <vilib>:"WPI_MotorControlRefNum Registry Get.vi"("refnum name"="disparador") -> ("error out"=w283:errorcluster, "MotorControlDevRef"=w282:T3)  [unwired: 9 in]
                n166 = call <vilib>:"WPI_MotorControlSetOutput.vi"("error in (no error)"=w281, "Output"=0.0, "MotorControlDevRef"=w280) -> ()  [unwired: 6 in, 3 out]
                n167 = call <vilib>:"WPI_MotorControlSetOutput.vi"("error in (no error)"=w283, "Output"=0.0, "MotorControlDevRef"=w282) -> ()  [unwired: 6 in, 3 out]
              }
              frame #6 {
              }
            }
          }
          frame 2 {
            n168 = flat-sequence {
              tunnel: [3.0] -> w285
              frame #0 {
                n169 = call <vilib>:"WPI_RobotDriveRefNum Registry Get.vi"("refnum name"="chasis") -> ("error out"=w293:errorcluster, "RobotDriveDevRef"=w292:T8)  [unwired: 9 in]
                n170 = call-poly <vilib>:"NT Read Value.vi"("Name"="wait3") -> ("Numeric"=w286:dbl)  [unwired: 9 in, 1 out]
                n171 = call <vilib>:"WPI_RobotDriveTankDrive.vi"("error in (no error)"=w293, "Right axis value"=1.0, "Left axis value"=-1.0, "RobotDriveDevRef"=w292) -> ("RobotDriveDevRef"=w287:T8)  [unwired: 5 in, 2 out]
                n172 = call <vilib>:"WPI_RobotDriveDelayAndUpdateSafety.vi"("Delay (s)"=w286, "RobotDriveDevRef"=w287) -> ()  [unwired: 8 in, 2 out]
              }
              frame #1 {
                w294 = 0.0
                n173 = call <vilib>:"WPI_RobotDriveRefNum Registry Get.vi"("refnum name"="chasis") -> ("error out"=w295:errorcluster, "RobotDriveDevRef"=w296:T8)  [unwired: 9 in]
                n174 = call <vilib>:"WPI_RobotDriveTankDrive.vi"("error in (no error)"=w295, "Right axis value"=w294, "Left axis value"=w294, "RobotDriveDevRef"=w296) -> ()  [unwired: 5 in, 3 out]
              }
              frame #2 {
              }
            }
          }
          frame 3 {
            n175 = flat-sequence {
              tunnel: [4.0] -> w299
              frame #0 {
                n176 = while {
                  stop <- w305 stop-if-true
                  n177 = global read "Robot Global Data.vi" "cent"() -> (w306:bool)
                  n178 = global read "Robot Global Data.vi" "intake"() -> (w303:bool)
                  n179 = global read "Robot Global Data.vi" "der"() -> (w317:bool)
                  n180 = global read "Robot Global Data.vi" "izq"() -> (w318:bool)
                  n181 = Build Array(w318, w317, w306) -> (w316:bool[])
                  n182 = case shown="True" w303 {
                    tunnel: [0.0 -0.9] -> w311
                    frame False {
                    }
                    frame True {
                    }
                  }
                  n183 = Boolean Array To Number(Boolean array=w316) -> (number=w315:u32)
                  n184 = case shown="1" w315 {
                    tunnel: [w321 0.5 -0.5 w326] -> w301
                    tunnel: [w321 -0.5 0.5 w326] -> w300
                    frame 0, Default {
                      w321 = -0.5
                    }
                    frame 1 {
                    }
                    frame 2 {
                    }
                    frame 4 {
                      w326 = -0.5
                    }
                  }
                  n185 = global read "Robot Global Data.vi" "y"() -> (w304:dbl)
                  n186 = call-poly <vilib>:"NT Read Value.vi"("Name"="ranky") -> ("Numeric"=w302:dbl)  [unwired: 9 in, 1 out]
                  n187 = call <vilib>:"WPI_MotorControlRefNum Registry Get.vi"("refnum name"="intake") -> ("error out"=w309:errorcluster, "MotorControlDevRef"=w310:T3)  [unwired: 9 in]
                  n188 = call <vilib>:"WPI_MotorControlSetOutput.vi"("error in (no error)"=w309, "Output"=w311, "MotorControlDevRef"=w310) -> ()  [unwired: 6 in, 3 out]
                  n189 = Greater?(x=w304, y=w302) -> (0:w305:bool)
                  n190 = call <vilib>:"WPI_RobotDriveRefNum Registry Get.vi"("refnum name"="chasis") -> ("error out"=w313:errorcluster, "RobotDriveDevRef"=w314:T8)  [unwired: 9 in]
                  n191 = call <vilib>:"WPI_RobotDriveTankDrive.vi"("error in (no error)"=w313, "Right axis value"=w300, "Left axis value"=w301, "RobotDriveDevRef"=w314) -> ()  [unwired: 5 in, 3 out]
                }
              }
              frame #1 {
                n192 = call <vilib>:"WPI_MotorControlRefNum Registry Get.vi"("refnum name"="intake") -> ("error out"=w330:errorcluster, "MotorControlDevRef"=w329:T3)  [unwired: 9 in]
                n193 = call <vilib>:"WPI_MotorControlSetOutput.vi"("error in (no error)"=w330, "Output"=-1.0, "MotorControlDevRef"=w329) -> ()  [unwired: 6 in, 3 out]
              }
              frame #2 {
                w335 = 0.7
                n194 = call <vilib>:"WPI_RobotDriveRefNum Registry Get.vi"("refnum name"="chasis") -> ("error out"=w336:errorcluster, "RobotDriveDevRef"=w337:T8)  [unwired: 9 in]
                n195 = call-poly <vilib>:"NT Read Value.vi"("Name"="wait3") -> ("Numeric"=w333:dbl)  [unwired: 9 in, 1 out]
                n196 = call <vilib>:"WPI_RobotDriveTankDrive.vi"("error in (no error)"=w336, "Right axis value"=w335, "Left axis value"=w335, "RobotDriveDevRef"=w337) -> ("error out"=w331:errorcluster, "RobotDriveDevRef"=w332:T8)  [unwired: 5 in, 1 out]
                n197 = call <vilib>:"WPI_RobotDriveDelayAndUpdateSafety.vi"("error in (no error)"=w331, "Delay (s)"=w333, "RobotDriveDevRef"=w332) -> ()  [unwired: 7 in, 2 out]
              }
              frame #3 {
                n198 = call <vilib>:"WPI_MotorControlRefNum Registry Get.vi"("refnum name"="intake") -> ("error out"=w341:errorcluster, "MotorControlDevRef"=w342:T3)  [unwired: 9 in]
                n199 = call <vilib>:"WPI_MotorControlSetOutput.vi"("error in (no error)"=w341, "Output"=0.0, "MotorControlDevRef"=w342) -> ()  [unwired: 6 in, 3 out]
              }
              frame #4 {
              }
            }
          }
          frame 4 {
            n200 = flat-sequence {
              tunnel: [5.0] -> w344
              frame #0 {
                n201 = call-poly <vilib>:"NT Read Value.vi"("Name"="wait4") -> ("Numeric"=w347:dbl)  [unwired: 9 in, 1 out]
                n202 = Multiply(x=1000.0, y=w347) -> (x*y=w346:dbl)
                n203 = Wait (ms)(milliseconds to wait=w346) -> ()  [unwired: 1 out]
              }
              frame #1 {
                n204 = while {
                  stop <- w350 stop-if-true
                  n205 = global read "Robot Global Data.vi" "cent"() -> (w349:bool)
                  n206 = global read "Robot Global Data.vi" "izq"() -> (w356:bool)
                  n207 = call <vilib>:"WPI_RobotDriveRefNum Registry Get.vi"("refnum name"="chasis") -> ("error out"=w353:errorcluster, "RobotDriveDevRef"=w354:T8)  [unwired: 9 in]
                  n208 = Compound Arithmetic op=OR(w356, w349) -> (w350:bool)
                  n209 = call <vilib>:"WPI_RobotDriveTankDrive.vi"("error in (no error)"=w353, "Right axis value"=0.5, "Left axis value"=-0.5, "RobotDriveDevRef"=w354) -> ()  [unwired: 5 in, 3 out]
                }
              }
              frame #2 {
                w357 = 0.0 ("Left axis value")
                n210 = call <vilib>:"WPI_RobotDriveRefNum Registry Get.vi"("refnum name"="chasis") -> ("error out"=w358:errorcluster, "RobotDriveDevRef"=w359:T8)  [unwired: 9 in]
                n211 = call <vilib>:"WPI_RobotDriveTankDrive.vi"("error in (no error)"=w358, "Right axis value"=w357, "Left axis value"=w357, "RobotDriveDevRef"=w359) -> ()  [unwired: 5 in, 3 out]
              }
              frame #3 {
              }
            }
          }
          frame 5 {
            n212 = flat-sequence {
              tunnel: [6.0] -> w362
              frame #0 {
                n213 = while {
                  stop <- w366 stop-if-true
                  n214 = global read "Robot Global Data.vi" "cent"() -> (w367:bool)
                  n215 = global read "Robot Global Data.vi" "der"() -> (w380:bool)
                  n216 = global read "Robot Global Data.vi" "izq"() -> (w381:bool)
                  n217 = Build Array(w381, w380, w367) -> (w379:bool[])
                  n218 = global read "Robot Global Data.vi" "intake"() -> (w364:bool)
                  n219 = global read "Robot Global Data.vi" "y"() -> (w365:dbl)
                  n220 = call-poly <vilib>:"NT Read Value.vi"("Name"="ranky") -> ("Numeric"=w363:dbl)  [unwired: 9 in, 1 out]
                  n221 = Boolean Array To Number(Boolean array=w379) -> (number=w378:u32)
                  n222 = case shown="4" w378 {
                    tunnel: [-0.5 0.5 -0.5 w390] -> w374
                    tunnel: [-0.5 -0.5 0.5 w390] -> w373
                    frame 0, Default {
                    }
                    frame 1 {
                    }
                    frame 2 {
                    }
                    frame 4 {
                      w390 = -0.5
                    }
                  }
                  n223 = Greater?(x=w365, y=w363) -> (0:w366:bool)
                  n224 = case shown="True" w364 {
                    tunnel: [0.0 -0.9] -> w372
                    frame False {
                    }
                    frame True {
                    }
                  }
                  n225 = call <vilib>:"WPI_MotorControlRefNum Registry Get.vi"("refnum name"="intake") -> ("error out"=w370:errorcluster, "MotorControlDevRef"=w371:T3)  [unwired: 9 in]
                  n226 = call <vilib>:"WPI_RobotDriveRefNum Registry Get.vi"("refnum name"="chasis") -> ("error out"=w376:errorcluster, "RobotDriveDevRef"=w377:T8)  [unwired: 9 in]
                  n227 = call <vilib>:"WPI_MotorControlSetOutput.vi"("error in (no error)"=w370, "Output"=w372, "MotorControlDevRef"=w371) -> ()  [unwired: 6 in, 3 out]
                  n228 = call <vilib>:"WPI_RobotDriveTankDrive.vi"("error in (no error)"=w376, "Right axis value"=w373, "Left axis value"=w374, "RobotDriveDevRef"=w377) -> ()  [unwired: 5 in, 3 out]
                }
              }
              frame #1 {
                w395 = 0.0
                n229 = call <vilib>:"WPI_RobotDriveRefNum Registry Get.vi"("refnum name"="chasis") -> ("error out"=w396:errorcluster, "RobotDriveDevRef"=w397:T8)  [unwired: 9 in]
                n230 = call <vilib>:"WPI_MotorControlRefNum Registry Get.vi"("refnum name"="intake") -> ("error out"=w394:errorcluster, "MotorControlDevRef"=w393:T3)  [unwired: 9 in]
                n231 = call <vilib>:"WPI_RobotDriveTankDrive.vi"("error in (no error)"=w396, "Right axis value"=w395, "Left axis value"=w395, "RobotDriveDevRef"=w397) -> ()  [unwired: 5 in, 3 out]
                n232 = call <vilib>:"WPI_MotorControlSetOutput.vi"("error in (no error)"=w394, "Output"=-1.0, "MotorControlDevRef"=w393) -> ()  [unwired: 6 in, 3 out]
              }
              frame #2 {
                n233 = call-poly <vilib>:"NT Read Value.vi"("Name"="wait5") -> ("Numeric"=w401:dbl)  [unwired: 9 in, 1 out]
                n234 = Multiply(x=1000.0, y=w401) -> (x*y=w400:dbl)
                n235 = Wait (ms)(milliseconds to wait=w400) -> ()  [unwired: 1 out]
              }
              frame #3 {
                n236 = call <vilib>:"WPI_MotorControlRefNum Registry Get.vi"("refnum name"="intake") -> ("error out"=w405:errorcluster, "MotorControlDevRef"=w406:T3)  [unwired: 9 in]
                n237 = call <vilib>:"WPI_MotorControlSetOutput.vi"("error in (no error)"=w405, "Output"=0.0, "MotorControlDevRef"=w406) -> ()  [unwired: 6 in, 3 out]
              }
              frame #4 {
              }
            }
          }
          frame 6 {
            n238 = flat-sequence {
              tunnel: [7.0] -> w408
              frame #0 {
                w409 = 0.7 ("Left axis value")
                n239 = call <vilib>:"WPI_RobotDriveRefNum Registry Get.vi"("refnum name"="chasis") -> ("error out"=w415:errorcluster, "RobotDriveDevRef"=w414:T8)  [unwired: 9 in]
                n240 = call <vilib>:"WPI_RobotDriveTankDrive.vi"("error in (no error)"=w415, "Right axis value"=w409, "Left axis value"=w409, "RobotDriveDevRef"=w414) -> ("RobotDriveDevRef"=w411:T8)  [unwired: 5 in, 2 out]
                n241 = call-poly <vilib>:"NT Read Value.vi"("Name"="wait6") -> ("Numeric"=w410:dbl)  [unwired: 9 in, 1 out]
                n242 = call <vilib>:"WPI_RobotDriveDelayAndUpdateSafety.vi"("Delay (s)"=w410, "RobotDriveDevRef"=w411) -> ()  [unwired: 8 in, 2 out]
              }
              frame #1 {
                w416 = 0.0
                n243 = call <vilib>:"WPI_RobotDriveRefNum Registry Get.vi"("refnum name"="chasis") -> ("error out"=w417:errorcluster, "RobotDriveDevRef"=w418:T8)  [unwired: 9 in]
                n244 = call <vilib>:"WPI_RobotDriveTankDrive.vi"("error in (no error)"=w417, "Right axis value"=w416, "Left axis value"=w416, "RobotDriveDevRef"=w418) -> ()  [unwired: 5 in, 3 out]
              }
              frame #2 {
              }
            }
          }
          frame 7 {
            n245 = flat-sequence {
              tunnel: [8.0] -> w421
              frame #0 {
                n246 = call <vilib>:"WPI_RobotDriveRefNum Registry Get.vi"("refnum name"="chasis") -> ("error out"=w429:errorcluster, "RobotDriveDevRef"=w428:T8)  [unwired: 9 in]
                n247 = call-poly <vilib>:"NT Read Value.vi"("Name"="wait7") -> ("Numeric"=w424:dbl)  [unwired: 9 in, 1 out]
                n248 = call <vilib>:"WPI_RobotDriveTankDrive.vi"("error in (no error)"=w429, "Right axis value"=1.0, "Left axis value"=-1.0, "RobotDriveDevRef"=w428) -> ("RobotDriveDevRef"=w425:T8)  [unwired: 5 in, 2 out]
                n249 = call <vilib>:"WPI_RobotDriveDelayAndUpdateSafety.vi"("Delay (s)"=w424, "RobotDriveDevRef"=w425) -> ()  [unwired: 8 in, 2 out]
              }
              frame #1 {
                w430 = 0.0
                n250 = call <vilib>:"WPI_RobotDriveRefNum Registry Get.vi"("refnum name"="chasis") -> ("error out"=w431:errorcluster, "RobotDriveDevRef"=w432:T8)  [unwired: 9 in]
                n251 = call <vilib>:"WPI_RobotDriveTankDrive.vi"("error in (no error)"=w431, "Right axis value"=w430, "Left axis value"=w430, "RobotDriveDevRef"=w432) -> ()  [unwired: 5 in, 3 out]
              }
              frame #2 {
              }
            }
          }
          frame 8 {
            n252 = flat-sequence {
              tunnel: [9.0] -> w435
              frame #0 {
                w436 = -0.7 ("Left axis value")
                n253 = call <vilib>:"WPI_RobotDriveRefNum Registry Get.vi"("refnum name"="chasis") -> ("error out"=w442:errorcluster, "RobotDriveDevRef"=w441:T8)  [unwired: 9 in]
                n254 = call <vilib>:"WPI_RobotDriveTankDrive.vi"("error in (no error)"=w442, "Right axis value"=w436, "Left axis value"=w436, "RobotDriveDevRef"=w441) -> ("RobotDriveDevRef"=w438:T8)  [unwired: 5 in, 2 out]
                n255 = call-poly <vilib>:"NT Read Value.vi"("Name"="wait8") -> ("Numeric"=w437:dbl)  [unwired: 9 in, 1 out]
                n256 = call <vilib>:"WPI_RobotDriveDelayAndUpdateSafety.vi"("Delay (s)"=w437, "RobotDriveDevRef"=w438) -> ()  [unwired: 8 in, 2 out]
              }
              frame #1 {
                w443 = 0.0
                n257 = call <vilib>:"WPI_RobotDriveRefNum Registry Get.vi"("refnum name"="chasis") -> ("error out"=w444:errorcluster, "RobotDriveDevRef"=w445:T8)  [unwired: 9 in]
                n258 = call <vilib>:"WPI_RobotDriveTankDrive.vi"("error in (no error)"=w444, "Right axis value"=w443, "Left axis value"=w443, "RobotDriveDevRef"=w445) -> ()  [unwired: 5 in, 3 out]
              }
              frame #2 {
              }
            }
          }
          frame 9 {
            n259 = flat-sequence {
              tunnel: [10.0] -> w449
              tunnel: [TRUE] -> w448
              frame #0 {
                n260 = call <vilib>:"WPI_MotorControlRefNum Registry Get.vi"("refnum name"="disparador") -> ("error out"=w455:errorcluster, "MotorControlDevRef"=w454:T3)  [unwired: 9 in]
                n261 = call-poly <vilib>:"NT Read Value.vi"("Name"="dispi2") -> ("Numeric"=w451:dbl)  [unwired: 9 in, 1 out]
                n262 = Negate(x=w451) -> (-x=w450:dbl)
                n263 = call <vilib>:"WPI_MotorControlSetOutput.vi"("error in (no error)"=w455, "Output"=w450, "MotorControlDevRef"=w454) -> ()  [unwired: 6 in, 3 out]
              }
              frame #1 {
                n264 = call-poly <vilib>:"NT Read Value.vi"("Name"="wait9") -> ("Numeric"=w458:dbl)  [unwired: 9 in, 1 out]
                n265 = Multiply(x=w458, y=1000.0) -> (x*y=w459:dbl)
                n266 = Wait (ms)(milliseconds to wait=w459) -> ()  [unwired: 1 out]
              }
              frame #2 {
                n267 = call-poly <vilib>:"NT Read Value.vi"("Name"="dispi2") -> ("Numeric"=w461:dbl)  [unwired: 9 in, 1 out]
                n268 = call <vilib>:"WPI_MotorControlRefNum Registry Get.vi"("refnum name"="banda") -> ("error out"=w465:errorcluster, "MotorControlDevRef"=w464:T3)  [unwired: 9 in]
                n269 = call <vilib>:"WPI_MotorControlRefNum Registry Get.vi"("refnum name"="disparador") -> ("error out"=w469:errorcluster, "MotorControlDevRef"=w468:T3)  [unwired: 9 in]
                n270 = Negate(x=w461) -> (-x=w460:dbl)
                n271 = call <vilib>:"WPI_MotorControlSetOutput.vi"("error in (no error)"=w465, "Output"=1.0, "MotorControlDevRef"=w464) -> ()  [unwired: 6 in, 3 out]
                n272 = call <vilib>:"WPI_MotorControlSetOutput.vi"("error in (no error)"=w469, "Output"=w460, "MotorControlDevRef"=w468) -> ()  [unwired: 6 in, 3 out]
              }
              frame #3 {
                n273 = call-poly <vilib>:"NT Read Value.vi"("Name"="wait10") -> ("Numeric"=w473:dbl)  [unwired: 9 in, 1 out]
                n274 = Multiply(x=w473, y=1000.0) -> (x*y=w470:dbl)
                n275 = Wait (ms)(milliseconds to wait=w470) -> ()  [unwired: 1 out]
              }
              frame #4 {
                n276 = call <vilib>:"WPI_MotorControlRefNum Registry Get.vi"("refnum name"="banda") -> ("error out"=w479:errorcluster, "MotorControlDevRef"=w478:T3)  [unwired: 9 in]
                n277 = call <vilib>:"WPI_MotorControlRefNum Registry Get.vi"("refnum name"="disparador") -> ("error out"=w481:errorcluster, "MotorControlDevRef"=w480:T3)  [unwired: 9 in]
                n278 = call <vilib>:"WPI_MotorControlSetOutput.vi"("error in (no error)"=w479, "Output"=0.0, "MotorControlDevRef"=w478) -> ()  [unwired: 6 in, 3 out]
                n279 = call <vilib>:"WPI_MotorControlSetOutput.vi"("error in (no error)"=w481, "Output"=0.0, "MotorControlDevRef"=w480) -> ()  [unwired: 6 in, 3 out]
              }
              frame #5 {
              }
            }
          }
        }
      }
    }
    frame "Shoot" {
      n280 = while {
        shift-right: [w485] -> _
        shift-left: 1.0 -> [w487]
        stop <- w486 stop-if-true
        n281 = case shown="1" w487 {
          tunnel: [0.0 w489] -> w485
          tunnel: [_ w490] -> w486
          frame 0, Default {
          }
          frame 1 {
            n282 = flat-sequence {
              tunnel: [2.0] -> w489
              tunnel: [TRUE] -> w490
              frame #0 {
                n283 = while {
                  stop <- w491 stop-if-true
                  n284 = global read "Robot Global Data.vi" "dio"() -> (w492:bool)
                  n285 = call <vilib>:"WPI_MotorControlRefNum Registry Get.vi"("refnum name"="upintake") -> ("error out"=w495:errorcluster, "MotorControlDevRef"=w496:T3)  [unwired: 9 in]
                  n286 = Not(x=w492) -> (.not. x?=w491:bool)
                  n287 = call <vilib>:"WPI_MotorControlSetOutput.vi"("error in (no error)"=w495, "Output"=-1.0, "MotorControlDevRef"=w496) -> ()  [unwired: 6 in, 3 out]
                }
              }
              frame #1 {
                n288 = call <vilib>:"WPI_MotorControlRefNum Registry Get.vi"("refnum name"="disparador") -> ("error out"=w501:errorcluster, "MotorControlDevRef"=w500:T3)  [unwired: 9 in]
                n289 = call-poly <vilib>:"NT Read Value.vi"("Name"="dispi1") -> ("Numeric"=w498:dbl)  [unwired: 9 in, 1 out]
                n290 = call <vilib>:"WPI_MotorControlSetOutput.vi"("error in (no error)"=w501, "Output"=w498, "MotorControlDevRef"=w500) -> ()  [unwired: 6 in, 3 out]
              }
              frame #2 {
                n291 = call-poly <vilib>:"NT Read Value.vi"("Name"="wait2") -> ("Numeric"=w505:dbl)  [unwired: 9 in, 1 out]
                n292 = Multiply(x=w505, y=1000.0) -> (x*y=w504:dbl)
                n293 = Wait (ms)(milliseconds to wait=w504) -> ()  [unwired: 1 out]
              }
              frame #3 {
                n294 = call <vilib>:"WPI_MotorControlRefNum Registry Get.vi"("refnum name"="banda") -> ("error out"=w509:errorcluster, "MotorControlDevRef"=w508:T3)  [unwired: 9 in]
                n295 = call <vilib>:"WPI_MotorControlRefNum Registry Get.vi"("refnum name"="disparador") -> ("error out"=w514:errorcluster, "MotorControlDevRef"=w513:T3)  [unwired: 9 in]
                n296 = call-poly <vilib>:"NT Read Value.vi"("Name"="dispi1") -> ("Numeric"=w511:dbl)  [unwired: 9 in, 1 out]
                n297 = call <vilib>:"WPI_MotorControlSetOutput.vi"("error in (no error)"=w509, "Output"=1.0, "MotorControlDevRef"=w508) -> ()  [unwired: 6 in, 3 out]
                n298 = call <vilib>:"WPI_MotorControlSetOutput.vi"("error in (no error)"=w514, "Output"=w511, "MotorControlDevRef"=w513) -> ()  [unwired: 6 in, 3 out]
              }
              frame #4 {
                n299 = call-poly <vilib>:"NT Read Value.vi"("Name"="wait3") -> ("Numeric"=w517:dbl)  [unwired: 9 in, 1 out]
                n300 = Multiply(x=w517, y=1000.0) -> (x*y=w518:dbl)
                n301 = Wait (ms)(milliseconds to wait=w518) -> ()  [unwired: 1 out]
              }
              frame #5 {
                n302 = call <vilib>:"WPI_MotorControlRefNum Registry Get.vi"("refnum name"="banda") -> ("error out"=w525:errorcluster, "MotorControlDevRef"=w526:T3)  [unwired: 9 in]
                n303 = call <vilib>:"WPI_MotorControlRefNum Registry Get.vi"("refnum name"="disparador") -> ("error out"=w523:errorcluster, "MotorControlDevRef"=w524:T3)  [unwired: 9 in]
                n304 = call <vilib>:"WPI_MotorControlSetOutput.vi"("error in (no error)"=w525, "Output"=0.0, "MotorControlDevRef"=w526) -> ()  [unwired: 6 in, 3 out]
                n305 = call <vilib>:"WPI_MotorControlSetOutput.vi"("error in (no error)"=w523, "Output"=0.0, "MotorControlDevRef"=w524) -> ()  [unwired: 6 in, 3 out]
              }
              frame #6 {
              }
            }
          }
        }
      }
    }
    frame "Shoot-Track" {
      n306 = while {
        shift-right: [w531] -> _
        shift-left: 1.0 -> [w532]
        stop <- w530 stop-if-true
        n307 = case shown="1" w532 {
          tunnel: [0.0 w534 w572] -> w531
          tunnel: [_ _ w573] -> w530
          frame 0, Default {
          }
          frame 1 {
            n308 = flat-sequence {
              tunnel: [2.0] -> w534
              frame #0 {
                n309 = while {
                  stop <- w535 stop-if-true
                  n310 = global read "Robot Global Data.vi" "dio"() -> (w536:bool)
                  n311 = call <vilib>:"WPI_MotorControlRefNum Registry Get.vi"("refnum name"="upintake") -> ("error out"=w539:errorcluster, "MotorControlDevRef"=w540:T3)  [unwired: 9 in]
                  n312 = Not(x=w536) -> (.not. x?=w535:bool)
                  n313 = call <vilib>:"WPI_MotorControlSetOutput.vi"("error in (no error)"=w539, "Output"=-1.0, "MotorControlDevRef"=w540) -> ()  [unwired: 6 in, 3 out]
                }
              }
              frame #1 {
                n314 = call <vilib>:"WPI_MotorControlRefNum Registry Get.vi"("refnum name"="disparador") -> ("error out"=w545:errorcluster, "MotorControlDevRef"=w544:T3)  [unwired: 9 in]
                n315 = call-poly <vilib>:"NT Read Value.vi"("Name"="dispi1") -> ("Numeric"=w542:dbl)  [unwired: 9 in, 1 out]
                n316 = call <vilib>:"WPI_MotorControlSetOutput.vi"("error in (no error)"=w545, "Output"=w542, "MotorControlDevRef"=w544) -> ()  [unwired: 6 in, 3 out]
              }
              frame #2 {
                n317 = call-poly <vilib>:"NT Read Value.vi"("Name"="wait2") -> ("Numeric"=w548:dbl)  [unwired: 9 in, 1 out]
                n318 = Multiply(x=w548, y=1000.0) -> (x*y=w549:dbl)
                n319 = Wait (ms)(milliseconds to wait=w549) -> ()  [unwired: 1 out]
              }
              frame #3 {
                n320 = call <vilib>:"WPI_MotorControlRefNum Registry Get.vi"("refnum name"="banda") -> ("error out"=w553:errorcluster, "MotorControlDevRef"=w552:T3)  [unwired: 9 in]
                n321 = call <vilib>:"WPI_MotorControlRefNum Registry Get.vi"("refnum name"="disparador") -> ("error out"=w558:errorcluster, "MotorControlDevRef"=w557:T3)  [unwired: 9 in]
                n322 = call-poly <vilib>:"NT Read Value.vi"("Name"="dispi1") -> ("Numeric"=w555:dbl)  [unwired: 9 in, 1 out]
                n323 = call <vilib>:"WPI_MotorControlSetOutput.vi"("error in (no error)"=w553, "Output"=1.0, "MotorControlDevRef"=w552) -> ()  [unwired: 6 in, 3 out]
                n324 = call <vilib>:"WPI_MotorControlSetOutput.vi"("error in (no error)"=w558, "Output"=w555, "MotorControlDevRef"=w557) -> ()  [unwired: 6 in, 3 out]
              }
              frame #4 {
                n325 = call-poly <vilib>:"NT Read Value.vi"("Name"="wait3") -> ("Numeric"=w562:dbl)  [unwired: 9 in, 1 out]
                n326 = Multiply(x=w562, y=1000.0) -> (x*y=w561:dbl)
                n327 = Wait (ms)(milliseconds to wait=w561) -> ()  [unwired: 1 out]
              }
              frame #5 {
                n328 = call <vilib>:"WPI_MotorControlRefNum Registry Get.vi"("refnum name"="banda") -> ("error out"=w569:errorcluster, "MotorControlDevRef"=w570:T3)  [unwired: 9 in]
                n329 = call <vilib>:"WPI_MotorControlRefNum Registry Get.vi"("refnum name"="disparador") -> ("error out"=w567:errorcluster, "MotorControlDevRef"=w568:T3)  [unwired: 9 in]
                n330 = call <vilib>:"WPI_MotorControlSetOutput.vi"("error in (no error)"=w569, "Output"=0.0, "MotorControlDevRef"=w570) -> ()  [unwired: 6 in, 3 out]
                n331 = call <vilib>:"WPI_MotorControlSetOutput.vi"("error in (no error)"=w567, "Output"=0.0, "MotorControlDevRef"=w568) -> ()  [unwired: 6 in, 3 out]
              }
              frame #6 {
              }
            }
          }
          frame 2 {
            n332 = flat-sequence {
              tunnel: [3.0] -> w572
              tunnel: [TRUE] -> w573
              frame #0 {
                n333 = while {
                  stop <- w575 stop-if-true
                  n334 = global read "Robot Global Data.vi" "cent"() -> (w581:bool)
                  n335 = global read "Robot Global Data.vi" "izq"() -> (w574:bool)
                  n336 = Compound Arithmetic op=OR(w574, w581) -> (w575:bool)
                  n337 = call <vilib>:"WPI_RobotDriveRefNum Registry Get.vi"("refnum name"="chasis") -> ("error out"=w578:errorcluster, "RobotDriveDevRef"=w579:T8)  [unwired: 9 in]
                  n338 = call <vilib>:"WPI_RobotDriveTankDrive.vi"("error in (no error)"=w578, "Right axis value"=-1.0, "Left axis value"=1.0, "RobotDriveDevRef"=w579) -> ()  [unwired: 5 in, 3 out]
                }
              }
              frame #1 {
                n339 = while {
                  stop <- w584 stop-if-true
                  n340 = global read "Robot Global Data.vi" "der"() -> (w594:bool)
                  n341 = global read "Robot Global Data.vi" "izq"() -> (w595:bool)
                  n342 = global read "Robot Global Data.vi" "cent"() -> (w585:bool)
                  n343 = Build Array(w595, w594, w585) -> (w593:bool[])
                  n344 = Boolean Array To Number(Boolean array=w593) -> (number=w592:u32)
                  n345 = global read "Robot Global Data.vi" "y"() -> (w583:dbl)
                  n346 = call-poly <vilib>:"NT Read Value.vi"("Name"="ranky") -> ("Numeric"=w582:dbl)  [unwired: 9 in, 1 out]
                  n347 = Greater?(x=w583, y=w582) -> (0:w584:bool)
                  n348 = case shown="1" w592 {
                    tunnel: [-0.5 0.0 -0.5 w602] -> w588
                    tunnel: [-0.5 -0.5 0.0 w602] -> w587
                    frame 0, Default {
                    }
                    frame 1 {
                    }
                    frame 2 {
                    }
                    frame 4 {
                      w602 = -0.5
                    }
                  }
                  n349 = call <vilib>:"WPI_RobotDriveRefNum Registry Get.vi"("refnum name"="chasis") -> ("error out"=w590:errorcluster, "RobotDriveDevRef"=w591:T8)  [unwired: 9 in]
                  n350 = call <vilib>:"WPI_RobotDriveTankDrive.vi"("error in (no error)"=w590, "Right axis value"=w587, "Left axis value"=w588, "RobotDriveDevRef"=w591) -> ()  [unwired: 5 in, 3 out]
                }
              }
              frame #2 {
                w603 = 0.0
                n351 = call <vilib>:"WPI_RobotDriveRefNum Registry Get.vi"("refnum name"="chasis") -> ("error out"=w604:errorcluster, "RobotDriveDevRef"=w605:T8)  [unwired: 9 in]
                n352 = call <vilib>:"WPI_RobotDriveTankDrive.vi"("error in (no error)"=w604, "Right axis value"=w603, "Left axis value"=w603, "RobotDriveDevRef"=w605) -> ()  [unwired: 5 in, 3 out]
              }
              frame #3 {
              }
            }
          }
        }
      }
    }
    frame "Track" {
      n353 = flat-sequence {
        frame #0 {
          n354 = while {
            stop <- w609 stop-if-true
            n355 = call <vilib>:"WPI_MotorControlRefNum Registry Get.vi"("refnum name"="upintake") -> ("error out"=w613:errorcluster, "MotorControlDevRef"=w614:T3)  [unwired: 9 in]
            n356 = global read "Robot Global Data.vi" "dio"() -> (w610:bool)
            n357 = call <vilib>:"WPI_MotorControlSetOutput.vi"("error in (no error)"=w613, "Output"=-1.0, "MotorControlDevRef"=w614) -> ()  [unwired: 6 in, 3 out]
            n358 = Not(x=w610) -> (.not. x?=w609:bool)
          }
        }
        frame #1 {
          n359 = while {
            stop <- FALSE stop-if-true
            n360 = global read "Robot Global Data.vi" "cent"() -> (w619:bool)
            n361 = global read "Robot Global Data.vi" "der"() -> (w628:bool)
            n362 = global read "Robot Global Data.vi" "izq"() -> (w629:bool)
            n363 = global read "Robot Global Data.vi" "y"() -> (w618:dbl)
            n364 = call-poly <vilib>:"NT Read Value.vi"("Name"="ranky") -> ("Numeric"=w617:dbl)  [unwired: 9 in, 1 out]
            n365 = Build Array(w629, w628, w619) -> (w627:bool[])
            n366 = Boolean Array To Number(Boolean array=w627) -> (number=w626:u32)
            n367 = Greater?(x=w618, y=w617) -> (0:w616:bool)
            n368 = case shown="4" w626 {
              tunnel: [0.6 0.6 0.6 w637] -> w622
              tunnel: [-0.6 -0.6 -0.6 w637] -> w621
              tunnel: w616 -> [_ _ _ w636]
              frame 0, Default {
              }
              frame 1 {
              }
              frame 2 {
              }
              frame 4 {
                n369 = case shown="True" w636 {
                  tunnel: [-0.6 0.0] -> w637
                  frame False {
                  }
                  frame True {
                  }
                }
              }
            }
            n370 = call <vilib>:"WPI_RobotDriveRefNum Registry Get.vi"("refnum name"="chasis") -> ("error out"=w624:errorcluster, "RobotDriveDevRef"=w625:T8)  [unwired: 9 in]
            n371 = call <vilib>:"WPI_RobotDriveTankDrive.vi"("error in (no error)"=w624, "Right axis value"=w621, "Left axis value"=w622, "RobotDriveDevRef"=w625) -> ()  [unwired: 5 in, 3 out]
          }
        }
      }
    }
    frame "Nothing" {
    }
  }
